vi "initJob.vi"(8 "error in (no error)":errorcluster, 10 "stdin":string, 11 "Job in":refnum<class "Job.lvclass">) -> (0 "error out":errorcluster, 3 "Job out":refnum<class "Job.lvclass">)   [LabVIEW 2013, in "openCronJob.lvlib" / "Job.lvclass"]
uses:
  Job.lvclass
  Job Details -- cluster.ctl
  Job.lvclass/Job.ctl
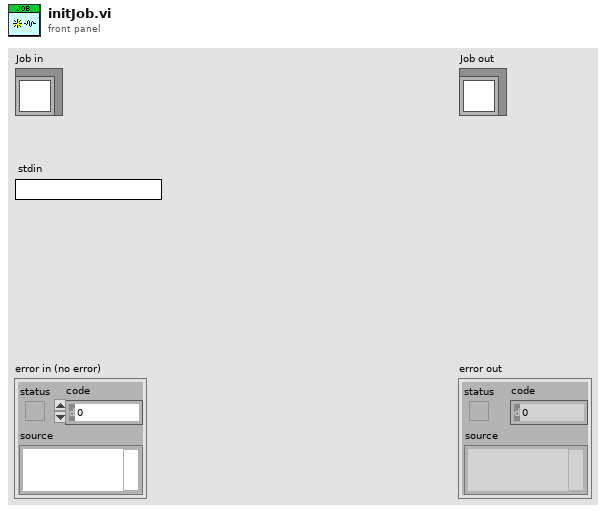
[diagram p1: front panel]
types:
  T1 = typedef "openCronJob.lvlib/Job.lvclass/Job Details -- cluster.ctl" = cluster{"Name":string, "GUID":string, "Abort":refnum<notifier>}
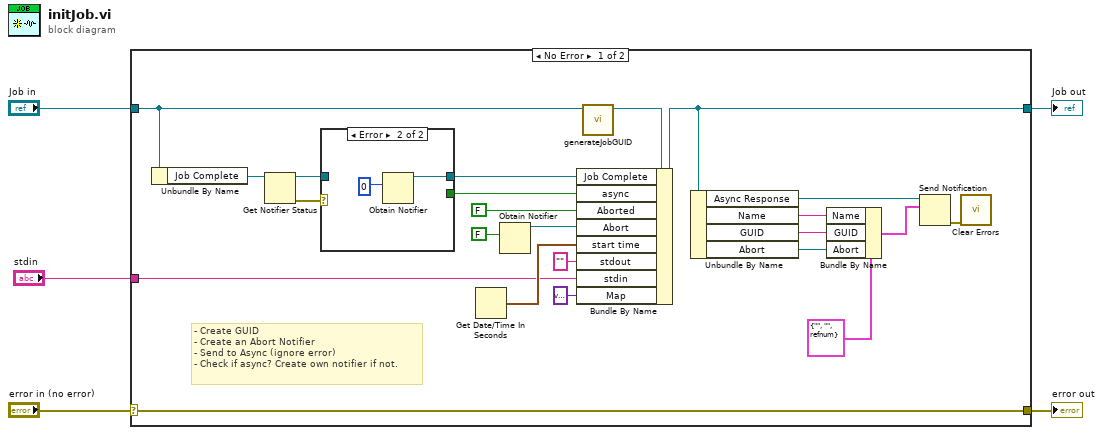
[diagram p0: block diagram]
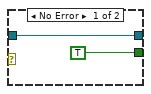
[diagram p2: hidden frame]
diagram:
  n1 = case shown="No Error" "error in (no error)" {
    selector: "error in (no error)" -> [w28 w34]
    tunnel: [w28 w34] -> w4
    tunnel: [w17 w33] -> w2
    tunnel: "Job in" -> [w15 w33]
    tunnel: "stdin" -> [w7 _]
    frame No Error {
      # "- Create GUID\n- Create an Abort Notifier\n- Send to Async (ignore error)\n- Check if async? Create own notifier if not."
      n2 = Unbundle By Name(w15) -> ("Job Complete"=w14:refnum<notifier>)
      n3 = Get Notifier Status(notifier=w14) -> (notifier out=w12:refnum<notifier>, error out=w13:errorcluster)  [unwired: 1 in, 3 out]
      n4 = case shown="Error" w13 {
        tunnel: w12 -> [w30 _]
        tunnel: [w30 w32] -> w11
        tunnel: [TRUE _] -> w10
        frame No Error {
        }
        frame Error {
          n5 = Obtain Notifier(notification data type=0) -> (notifier out=w32:refnum<notifier>)  [unwired: 3 in, 2 out]
        }
      }
      n6 = Get Date/Time In Seconds() -> (seconds since 1Jan1904=w8:timestamp)
      n7 = Obtain Notifier(notification data type=FALSE) -> (notifier out=w19:refnum<notifier>)  [unwired: 3 in, 2 out]
      n8 = call "generateJobGUID.vi"("Job in"=w15) -> ("Job out"=w18:refnum<class "Job.lvclass">)  [unwired: 9 in, 1 out]
      n9 = Bundle By Name(cluster=w18, "Job Complete"=w11, "async"=w10, "Aborted"=FALSE, "Abort"=w19, "start time"=w8, "stdout"="" ("stdin"), "stdin"=w7, "Map"=variant) -> (w17:refnum<class "Job.lvclass">)
      n10 = Unbundle By Name(w17) -> ("Async Response"=w27:refnum<notifier>, "Name"=w24:string, "GUID"=w23:string, "Abort"=w22:refnum<notifier>)
      n11 = Bundle By Name(cluster=T1 {"Name"="", "GUID"="", "Abort"=refnum} ("Job Details"), "Name"=w24, "GUID"=w23, "Abort"=w22) -> (w21:T1)
      n12 = Send Notification(notification=w21, notifier=w27) -> (error out=w26:errorcluster)  [unwired: 1 in, 1 out]
      n13 = call <vilib>:"Clear Errors.vi"("error in (no error)"=w26) -> ()  [unwired: 6 in, 1 out]
    }
    frame Error {
    }
  }
  "error out" <- w4
  "Job out" <- w2
